vi "updateSetting.vi"(8 "error in (no error)":errorcluster, 9 "Enum":T1(ring), 10 "Pane":refnum<vi>, 11 "ICSettingsViewer in":refnum<class "ICSettingsViewer.lvclass">) -> (0 "error out":errorcluster, 2 "Pane out":refnum<vi>, 3 "ICSettingsViewer out":refnum<class "ICSettingsViewer.lvclass">)   [LabVIEW 2009, in "Views.lvlib" / "Camera.lvlib" / "ICSettingsViewer.lvclass"]
uses:
  ICSettingsViewer.lvclass
  Tools/SettingsEventManager/SettingsEventsManager.lvclass
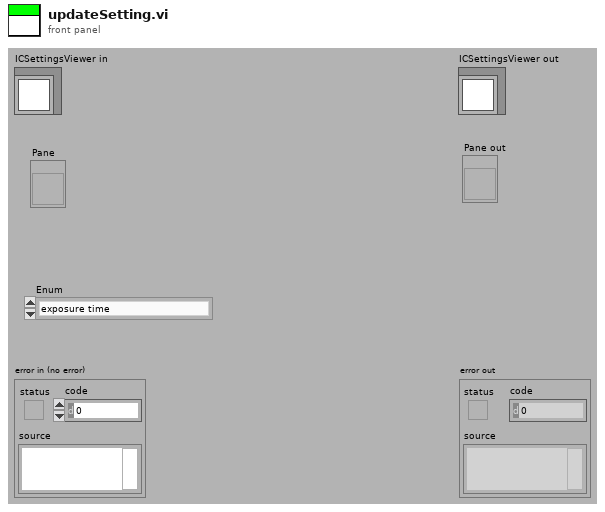
[diagram p1: front panel]
types:
  T1 = enum16{"exposure time", "gain", "trigger mode", "image number"}
  T2 = enum16{"exposure", "gain", "image_number", "Triggering"}
  T3 = cluster{"settingsFrontEndEvents":cluster{"loadSettingsFromPath":refnum<user-event>, "lookUpElementEvent":refnum<user-event>, "saveSettings":refnum<user-event>, "loadSettings":refnum<user-event>, "close":refnum<user-event>, "replaceElement":refnum<user-event>, "findParentNodes":refnum<user-event>, "createNode":refnum<user-event>}, "settingBackEndEvents":cluster{"defaultSettingsPathRequest":refnum<user-event>, "searchResultEvent":refnum<user-event>, "settingsSaved":refnum<user-event>, "settingsLoaded":refnum<user-event>, "foundParentNode":refnum<user-event>}}
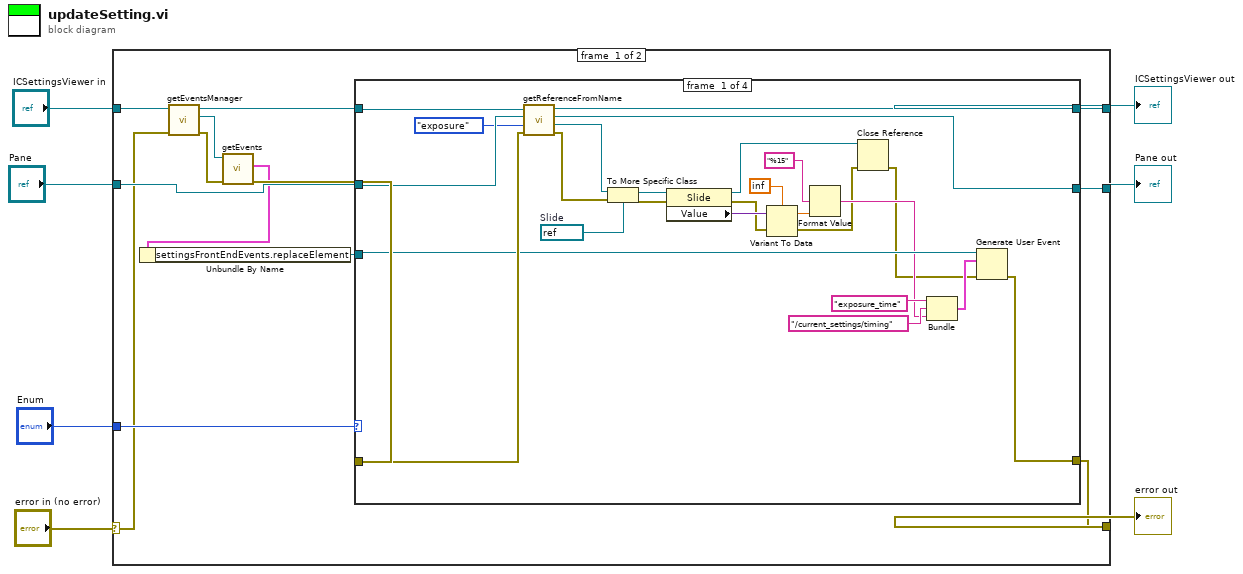
[diagram p0: block diagram]
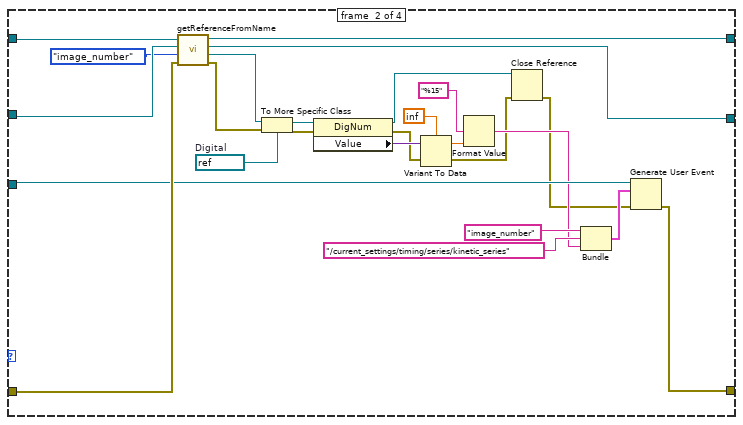
[diagram p2: hidden frame]
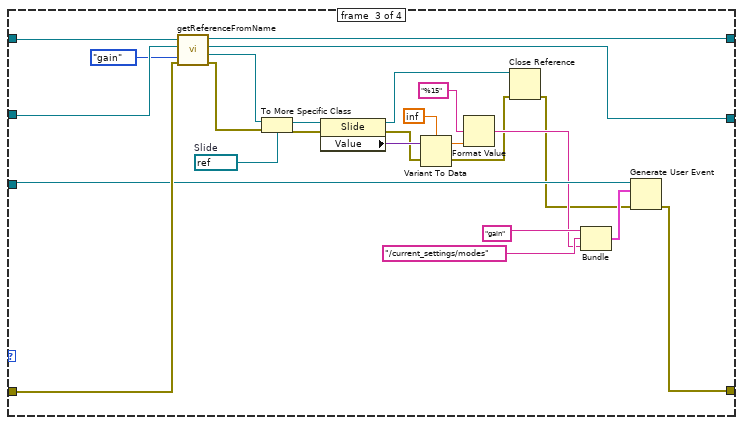
[diagram p3: hidden frame]
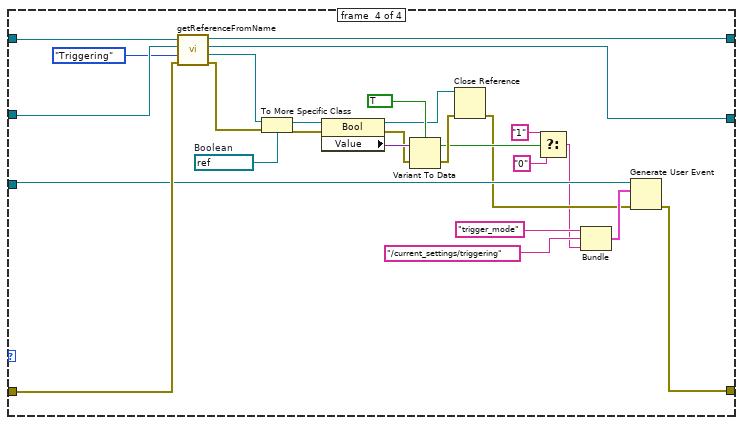
[diagram p4: hidden frame]
diagram:
  n1 = case shown="No Error" "error in (no error)" {
    selector: "error in (no error)" -> [w11 w123]
    tunnel: [w16 w123] -> w6
    tunnel: [w19 w122] -> w4
    tunnel: "ICSettingsViewer in" -> [w13 w122]
    tunnel: "Enum" -> [w20 _]
    tunnel: "Pane" -> [w18 _]
    tunnel: [w17 _] -> w1
    frame #0 {
      n2 = call-dynamic "getEventsManager.vi"("error in (no error)"=w11, "SettingsViewer.lvclass in"=w13) -> ("error out"=w14:errorcluster, "Tools.lvlib:Settings.lvlib:SettingsEventsManager.lvclass"=w15:refnum<class "SettingsEventsManager.lvclass">, "SettingsViewer.lvclass out"=w12:refnum<class "ICSettingsViewer.lvclass">)  [unwired: 7 in]
      n3 = call-dynamic "getEvents.vi"("error in (no error)"=w14, "SettingsEventsManager in"=w15) -> ("error out"=w10:errorcluster, "settingsEvents"=w9:T3)  [unwired: 7 in, 1 out]
      n4 = Unbundle By Name(w9) -> ("settingsFrontEndEvents.replaceElement"=w8:refnum<user-event>)
      n5 = case shown="\"trigger mode\"" w20 {
        tunnel: w12 -> [w45 w70 w95 w121]
        tunnel: [w44 w69 w94 w120] -> w19
        tunnel: w18 -> [w22 w67 w92 w97]
        tunnel: w10 -> [w43 w68 w93 w119]
        tunnel: [w42 w66 w91 w118] -> w17
        tunnel: [w26 w50 w75 w108] -> w16
        tunnel: w8 -> [w31 w55 w80 w112]
        frame #0 {
          w41 = refnum<vi> refnum  # Slide
          n6 = call "getReferenceFromName.vi"("error in (no error)"=w43, "referenceName"=T2."exposure", "Pane"=w22, "ICSettingsViewer in"=w45) -> ("error out"=w39:errorcluster, "Ctl Refnum"=w40:refnum<vi>, "Pane out"=w42:refnum<vi>, "ICSettingsViewer out"=w44:refnum<class "ICSettingsViewer.lvclass">)  [unwired: 3 in, 1 out]
          n7 = To More Specific Class(target class=w41, reference=w40, error in=w39) -> (specific class reference=w38:refnum<vi>, error out=w37:errorcluster)
          n8 = property class="Slide"(reference=w38, error in=w37) -> (reference out=w25:refnum<vi>, error out=w35:errorcluster, "Value"=w36:variant)
          n9 = Variant To Data(error in=w35, Variant=w36, type=inf) -> (error out=w24:errorcluster, data=w33:dbl)
          n10 = Format Value(format string="%15", value (0)=w33) -> (output string=w28:string)  [unwired: 1 in]
          n11 = Close Reference(reference=w25, error in (no error)=w24) -> (error out=w23:errorcluster)
          n12 = Bundle("exposure_time", "/current_settings/timing", "output string"=w28) -> (w27:cluster{string, string, "output string":string})  [unwired: 1 in]
          n13 = Generate User Event(user event=w31, event data cluster=w27, error in=w23) -> (error out=w26:errorcluster)  [unwired: 1 out]
        }
        frame #1 {
          w65 = refnum<vi> refnum  # Digital
          n14 = call "getReferenceFromName.vi"("error in (no error)"=w68, "referenceName"=T2."image_number", "Pane"=w67, "ICSettingsViewer in"=w70) -> ("error out"=w63:errorcluster, "Ctl Refnum"=w64:refnum<vi>, "Pane out"=w66:refnum<vi>, "ICSettingsViewer out"=w69:refnum<class "ICSettingsViewer.lvclass">)  [unwired: 3 in, 1 out]
          n15 = To More Specific Class(target class=w65, reference=w64, error in=w63) -> (specific class reference=w62:refnum<vi>, error out=w61:errorcluster)
          n16 = property class="DigNum"(reference=w62, error in=w61) -> (reference out=w49:refnum<vi>, error out=w59:errorcluster, "Value"=w60:variant)
          n17 = Variant To Data(error in=w59, Variant=w60, type=inf) -> (error out=w48:errorcluster, data=w57:dbl)
          n18 = Format Value(format string="%15", value (0)=w57) -> (output string=w52:string)  [unwired: 1 in]
          n19 = Close Reference(reference=w49, error in (no error)=w48) -> (error out=w47:errorcluster)
          n20 = Bundle("image_number", "/current_settings/timing/series/kinetic_series", "output string"=w52) -> (w51:cluster{string, string, "output string":string})  [unwired: 1 in]
          n21 = Generate User Event(user event=w55, event data cluster=w51, error in=w47) -> (error out=w50:errorcluster)  [unwired: 1 out]
        }
        frame #2 {
          w90 = refnum<vi> refnum  # Slide
          n22 = call "getReferenceFromName.vi"("error in (no error)"=w93, "referenceName"=T2."gain", "Pane"=w92, "ICSettingsViewer in"=w95) -> ("error out"=w88:errorcluster, "Ctl Refnum"=w89:refnum<vi>, "Pane out"=w91:refnum<vi>, "ICSettingsViewer out"=w94:refnum<class "ICSettingsViewer.lvclass">)  [unwired: 3 in, 1 out]
          n23 = To More Specific Class(target class=w90, reference=w89, error in=w88) -> (specific class reference=w87:refnum<vi>, error out=w86:errorcluster)
          n24 = property class="Slide"(reference=w87, error in=w86) -> (reference out=w74:refnum<vi>, error out=w84:errorcluster, "Value"=w85:variant)
          n25 = Variant To Data(error in=w84, Variant=w85, type=inf) -> (error out=w73:errorcluster, data=w82:dbl)
          n26 = Format Value(format string="%15", value (0)=w82) -> (output string=w77:string)  [unwired: 1 in]
          n27 = Close Reference(reference=w74, error in (no error)=w73) -> (error out=w72:errorcluster)
          n28 = Bundle("gain", "/current_settings/modes", "output string"=w77) -> (w76:cluster{string, string, "output string":string})  [unwired: 1 in]
          n29 = Generate User Event(user event=w80, event data cluster=w76, error in=w72) -> (error out=w75:errorcluster)  [unwired: 1 out]
        }
        frame #3 {
          w117 = refnum<vi> refnum  # Boolean
          n30 = call "getReferenceFromName.vi"("error in (no error)"=w119, "referenceName"=T2."Triggering", "Pane"=w97, "ICSettingsViewer in"=w121) -> ("error out"=w115:errorcluster, "Ctl Refnum"=w116:refnum<vi>, "Pane out"=w118:refnum<vi>, "ICSettingsViewer out"=w120:refnum<class "ICSettingsViewer.lvclass">)  [unwired: 3 in, 1 out]
          n31 = To More Specific Class(target class=w117, reference=w116, error in=w115) -> (specific class reference=w114:refnum<vi>, error out=w113:errorcluster)
          n32 = property class="Bool"(reference=w114, error in=w113) -> (reference out=w104:refnum<vi>, error out=w105:errorcluster, "Value"=w107:variant)
          n33 = Variant To Data(error in=w105, Variant=w107, type=TRUE) -> (error out=w103:errorcluster, data=w102:bool)
          n34 = Close Reference(reference=w104, error in (no error)=w103) -> (error out=w99:errorcluster)
          n35 = Select(t="1", s=w102, f="0") -> (s? t:f=w98:string)
          n36 = Bundle("trigger_mode", "/current_settings/triggering", w98) -> (w109:cluster{string, string, string})  [unwired: 1 in]
          n37 = Generate User Event(user event=w112, event data cluster=w109, error in=w99) -> (error out=w108:errorcluster)  [unwired: 1 out]
        }
      }
    }
    frame #1 {
    }
  }
  "error out" <- w6
  "ICSettingsViewer out" <- w4
  "Pane out" <- w1
